vi "Analys Chart.vi"(3 "error in (no error)":errorcluster, 4 "error wave in":cluster{"Array":dbl[], "Array":dbl[]}) -> ()   [LabVIEW 2019]
panel:
  out "error visual":cluster{"Array":dbl[], "Array":dbl[]}(graph)
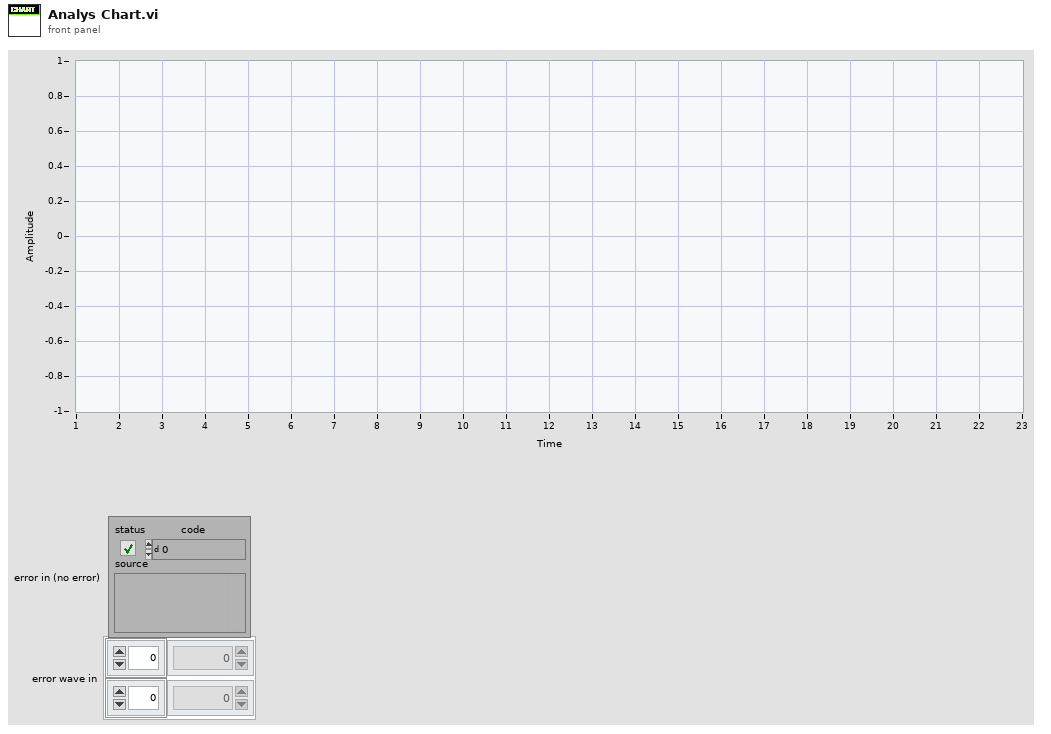
[diagram p1: front panel]
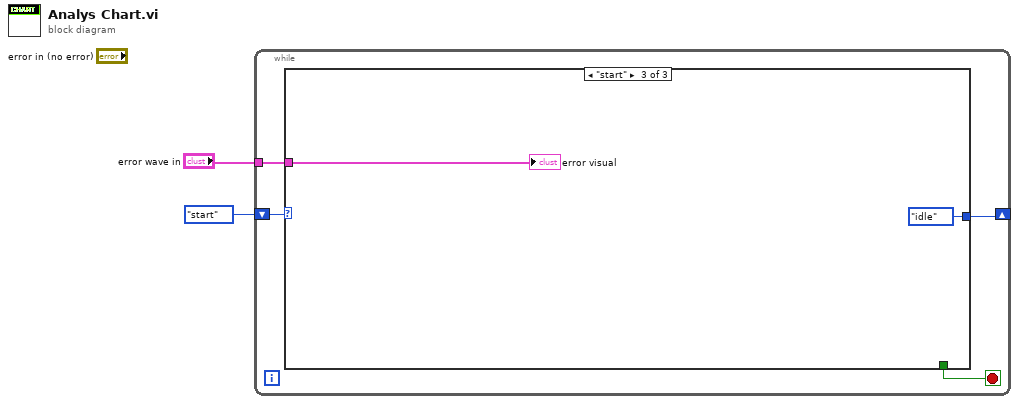
[diagram p0: block diagram]
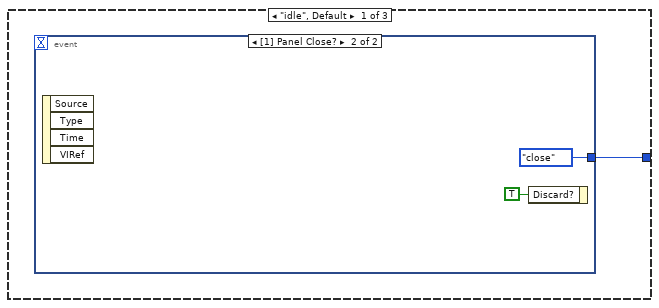
[diagram p2: hidden frame]
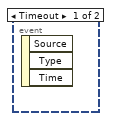
[diagram p3: hidden frame]
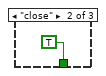
[diagram p4: hidden frame]
diagram:
  n1 = while {
    shift-right: [w5] -> _
    shift-left: enum16{"idle", "close", "start"}."start" -> [w6]
    tunnel: "error wave in" -> [w3]
    stop <- w4 stop-if-true
    n2 = case shown="\"start\"" w6 {
      tunnel: [w7 _ enum16{"idle", "close", "start"}."idle"] -> w5
      tunnel: [_ TRUE _] -> w4
      tunnel: w3 -> [_ _ w12]
      frame "idle", Default {
        n3 = event shown="[1] Panel Close?" {
          selector: _ -> [_ _]
          dyn-events: _ -> [_ _]
          timeout: _ -> [_ _]
          tunnel: [_ enum16{"idle", "close", "start"}."close"] -> w7
          event Timeout {
            n4 = event-data() -> ()  [unwired: 1 in, 3 out]
          }
          event Panel Close? {
            n5 = event-data() -> ()  [unwired: 1 in, 4 out]
            n6 = event-data("Discard?"=TRUE) -> ()  [unwired: 1 in, 1 out]
          }
        }
      }
      frame "close" {
      }
      frame "start" {
        "error visual" <- w12
      }
    }
  }
